vi "Fit.vi"(7 "Type X":T1(ring), 8 "error in (no error)":errorcluster caption="entrée d'erreur (pas d'erreur)", 9 "y":string[][](array[string]), 10 "X":string[][](array[string]), 11 "MaxAbsScaler.lvclass":refnum<class "MaxAbsScaler.lvclass">) -> (0 "error in (no error)":errorcluster caption="entrée d'erreur (pas d'erreur)", 2 "String Data":string, 3 "MaxAbsScaler.lvclass":refnum<class "MaxAbsScaler.lvclass">)   [LabVIEW 2020, in "MaxAbsScaler.lvclass"]
doc: "Compute the maximum absolute value to be used for later scaling.\n\nReturns : \n\n- String : OK"
uses:
  MaxAbsScaler.lvclass
  MaxAbsScaler.lvclass/MaxAbsScaler.ctl
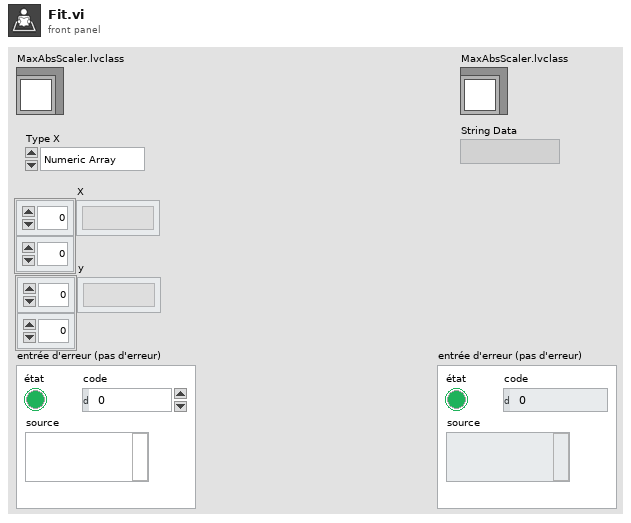
[diagram p1: front panel]
types:
  T1 = enum16{"Numeric Array", "String Array", "Sparse"}
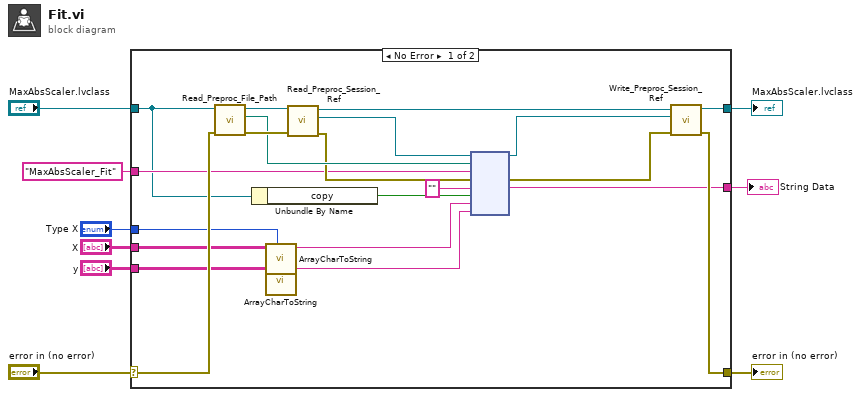
[diagram p0: block diagram]
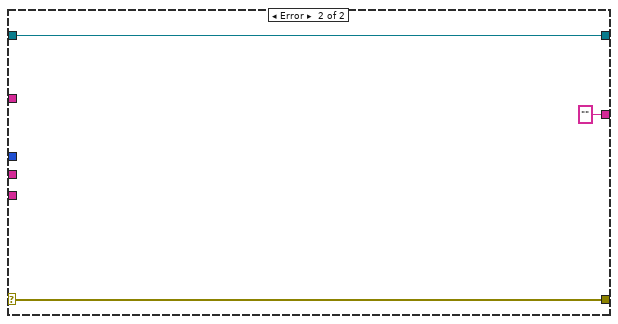
[diagram p2: hidden frame]
diagram:
  n1 = case shown="No Error" "error in (no error)" {
    selector: "error in (no error)" -> [w18 w33]
    tunnel: [w19 w33] -> w8
    tunnel: [w20 w32] -> w6
    tunnel: "MaxAbsScaler.lvclass" -> [w15 w32]
    tunnel: "MaxAbsScaler_Fit" ("Fonction") -> [w17 _]
    tunnel: [w16 ""] -> w4
    tunnel: "X" -> [w14 _]
    tunnel: "y" -> [w13 _]
    tunnel: "Type X" -> [w10 _]
    frame No Error {
      n2 = call-dynamic "Read_Preproc_File_Path.vi"("error in (no error)"=w18, "Python in"=w15) -> ("error out"=w29:errorcluster, "File_Path"=w26:path, "Python out"=w30:refnum<class "MaxAbsScaler.lvclass">)  [unwired: 7 in]
      n3 = Unbundle By Name(w15) -> ("copy"=w21:bool)
      n4 = call "ArrayCharToString.vi"("Type"=w10, "TAB"=w14) -> ("Instruction"=w12:string)  [unwired: 9 in]
      n5 = call "ArrayCharToString.vi"("TAB"=w13) -> ("Instruction"=w11:string)  [unwired: 10 in]
      n6 = call-dynamic "Read_Preproc_Session_Ref.vi"("error in (no error)"=w29, "Python in"=w30) -> ("error out"=w25:errorcluster, "Session_ref"=w27:refnum<k35>, "Python out"=w28:refnum<class "MaxAbsScaler.lvclass">)  [unwired: 7 in]
      n7 = node(w27, w26, w17, w25, "", w21, w12, w11) -> (w23:refnum<k35>, w24:errorcluster, w16:string)  [unwired: 3 in, 2 out]
      n8 = call-dynamic "Write_Preproc_Session_Ref.vi"("error in (no error)"=w24, "Session_ref"=w23, "Python in"=w28) -> ("error out"=w19:errorcluster, "Python out"=w20:refnum<class "MaxAbsScaler.lvclass">)  [unwired: 7 in]
    }
    frame Error {
    }
  }
  "error in (no error)" <- w8
  "MaxAbsScaler.lvclass" <- w6
  "String Data" <- w4
